vi "Class to gRPC_to_Main.vi"(11 "Timed Node in":refnum<class "ThermotronDriver.lvclass">) -> (2 "gRPC to Main":T1, 3 "Timed Node out":refnum<class "ThermotronDriver.lvclass">)   [LabVIEW 2023, in "ThermotronDriver.lvlib" / "ThermotronDriver.lvclass"]
uses:
  ThermotronDriver.lvclass
  Type Defs/gRPC to Main.ctl
  ThermotronDriver.lvclass/ThermotronDriver.ctl
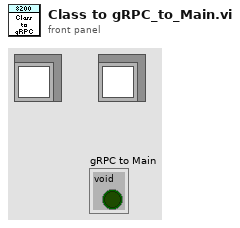
[diagram p1: front panel]
types:
  T1 = typedef "ThermotronDriver.lvlib/ThermotronDriver.lvclass/gRPC to Main.ctl" = cluster{"void":bool}
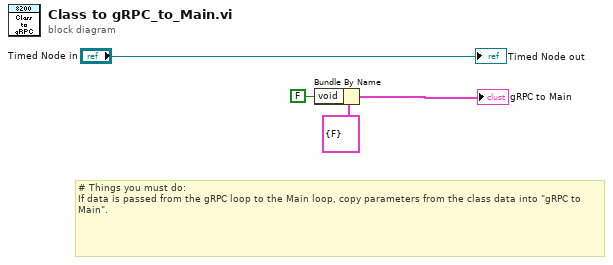
[diagram p0: block diagram]
diagram:
  # "# Things you must do:\nIf data is passed from the gRPC loop to the Main loop, copy parameters from the class data into \"gRPC to Main\"."
  n1 = Bundle By Name(cluster=T1 {"void"=FALSE} ("gRPC to Main"), "void"=FALSE) -> (→"gRPC to Main":T1)
  "Timed Node out" <- "Timed Node in"
